vi "checkBeginHaltPlay.vi"(8 "error in (no error)":errorcluster, 10 "Game":refnum<class "Game.lvclass">, 11 "HaltPlay in":refnum<class "HaltPlay.lvclass">) -> (0 "error out":errorcluster, 2 "Boolean":bool, 3 "HaltPlay out":refnum<class "HaltPlay.lvclass">)   [LabVIEW 2023, in "HaltPlay.lvclass"]
uses:
  HaltPlay.lvclass
  Game_class/Game.lvclass
  Referee_class/command_interpreted.ctl
  Game_class/Game.lvclass/Game.ctl
  Referee_class/Referee.lvclass/Referee.ctl
  Game_class/Read Referee.vi
  Referee_class/Read command_interpreted.vi
  Referee_class/Referee.lvclass
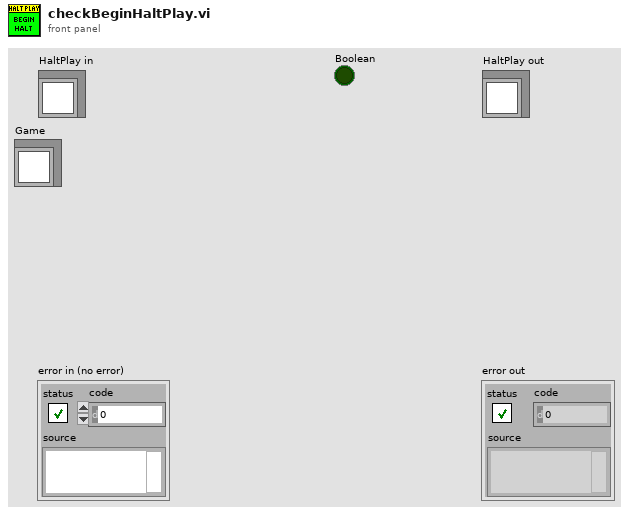
[diagram p1: front panel]
types:
  T1 = typedef "command_interpreted.ctl" = enum16{"Goal Ally", "Goal Enemy", "Ball Placement Enemy", "Ball Placement Ally", "Normal Half Time", "Extra Time  Break", "Extra Half Time", "None", "Post Game", "PKA Normal Start", "Prepare Kickoff Ally", "PKE Normal Start", "Prepare Kickoff Enemy", "Force Start", "Halt", "Timeout", "Prepare Penalty Ally", "Prepare Penalty Enemy", "PPA NormalStart", "PPE Normal Start", "Indirect Free Ally", "Direct Free Enemy", "Direct Free Ally", "Indirect Free Enemy", "Stop"}
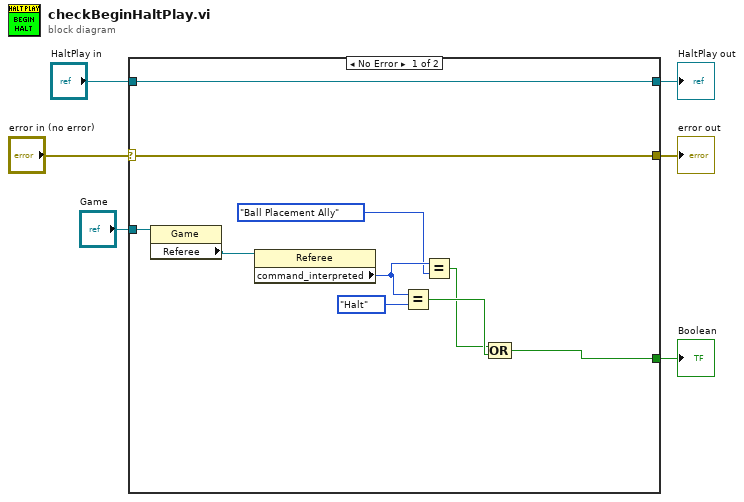
[diagram p0: block diagram]
diagram:
  n1 = case shown="No Error" "error in (no error)" {
    selector: "error in (no error)" -> [w15 w18]
    tunnel: [w15 w18] -> w5
    tunnel: [w16 w17] -> w3
    tunnel: "HaltPlay in" -> [w16 w17]
    tunnel: "Game" -> [w14 _]
    tunnel: [w12 _] -> w1
    frame No Error {
      n2 = property class="Game"(reference=w14) -> ("Referee"=w13:refnum<class "Referee.lvclass">)  [unwired: 1 in, 2 out]
      n3 = property class="Referee"(reference=w13) -> ("command_interpreted"=w9:T1)  [unwired: 1 in, 2 out]
      n4 = Equal?(x=w9, y=command_interpreted."Halt" ("command_interpreted")) -> (x = y?=w10:bool)
      n5 = Equal?(x=w9, y=command_interpreted."Ball Placement Ally" ("command_interpreted")) -> (x = y?=w7:bool)
      n6 = Compound Arithmetic op=OR(w7, w10) -> (w12:bool)
    }
    frame Error {
    }
  }
  "error out" <- w5
  "HaltPlay out" <- w3
  "Boolean" <- w1
